vi "FTW-Menu-DragDropDataAppend.vi"(3 "Data":variant, 4 "Name":string, 5 "Drag/Drop Data in":T1(array[cluster])) -> (2 "Drag/Drop Data":T1(array[cluster]))   [LabVIEW 2015]
panel:
  # "Inputs"
  # "Outputs"
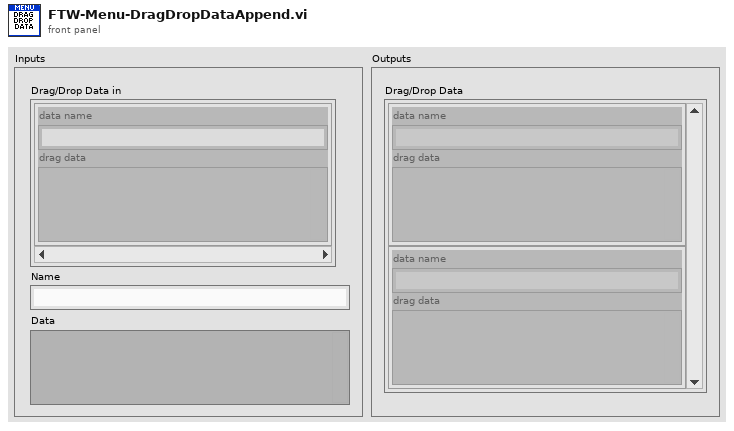
[diagram p1: front panel]
types:
  T1 = cluster{"data name":string, "drag data":variant}[]
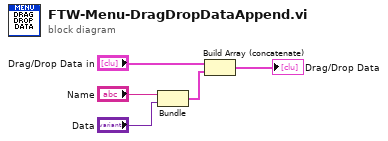
[diagram p0: block diagram]
diagram:
  n1 = Bundle("Name"="Name", "Data"="Data") -> (w2:cluster{"Name":string, "Data":variant})  [unwired: 1 in]
  n2 = Build Array (concatenate)("Drag/Drop Data in", w2) -> (→"Drag/Drop Data":cluster{"Name":string, "Data":variant}[])
